vi "CheckParameters.vi"(8 "error in (no error)":errorcluster, 10 "Parameters":u32[](array[numeric]), 11 "HF-Felder in":refnum<class "HF-Felder.lvclass">) -> (0 "error out":errorcluster, 3 "HF-Felder out":refnum<class "HF-Felder.lvclass">)   [LabVIEW 2013, in "HF-Felder.lvclass"]
uses:
  HF-Felder.lvclass
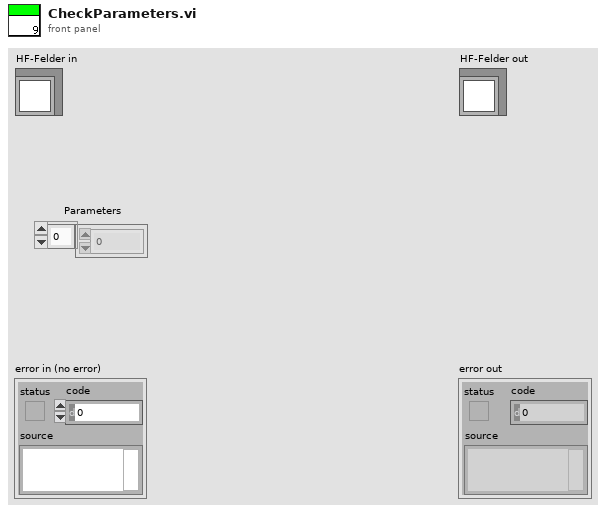
[diagram p1: front panel]
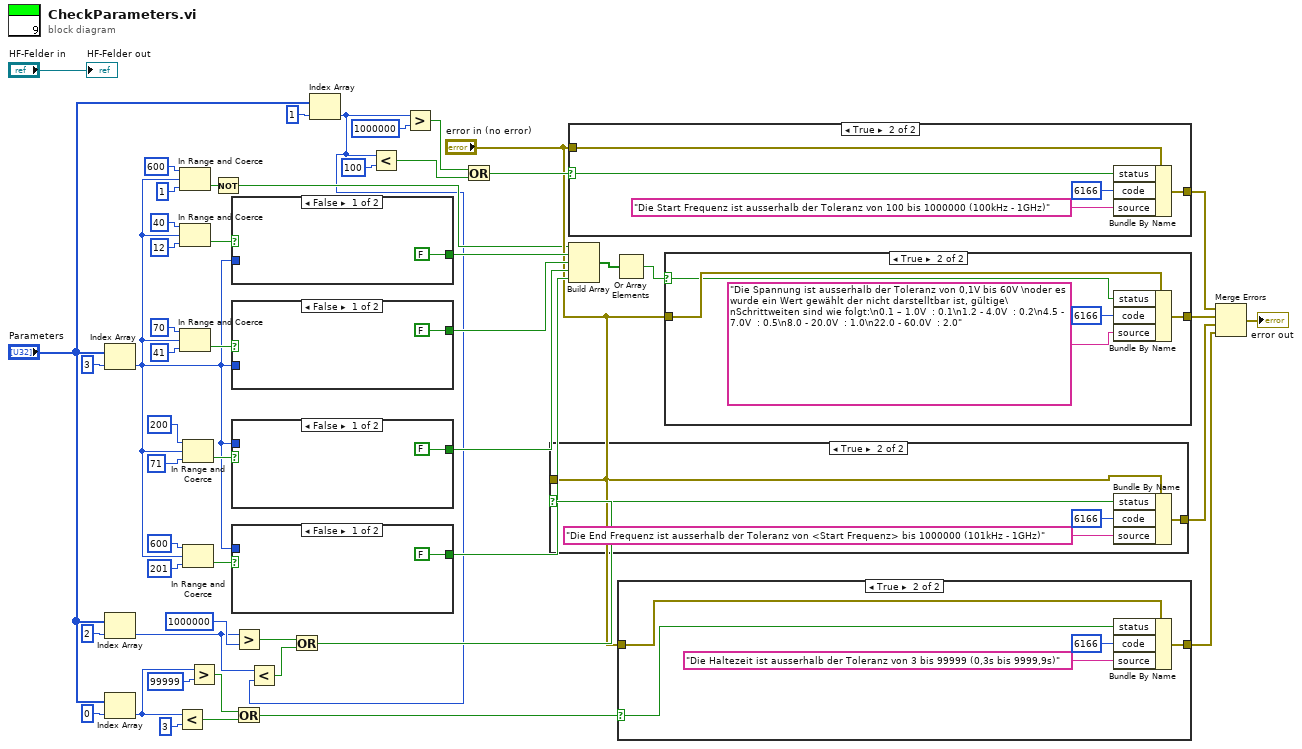
[diagram p0: block diagram]
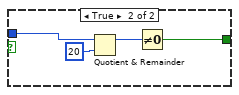
[diagram p2: hidden frame]
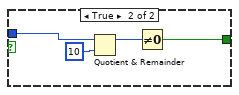
[diagram p3: hidden frame]
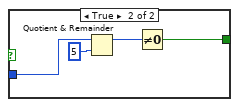
[diagram p4: hidden frame]
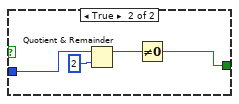
[diagram p5: hidden frame]
diagram:
  n1 = Index Array(array="Parameters", index=3) -> (element=w4:u32)
  n2 = Index Array(array="Parameters", index=2) -> (element=w30:u32)
  n3 = Index Array(array="Parameters", index=0) -> (element=w29:u32)
  n4 = Less?(x=w29, y=u32 3) -> (x < y?=w43:bool)
  n5 = In Range and Coerce(upper limit=u32 600 ("Obergrenze"), x=w4, lower limit=u32 1 ("Untergrenze")) -> (In Range?=w3:bool)  [unwired: 1 out]
  n6 = In Range and Coerce(upper limit=u32 40 ("Obergrenze"), x=w4, lower limit=u32 12 ("Untergrenze")) -> (In Range?=w21:bool)  [unwired: 1 out]
  n7 = In Range and Coerce(upper limit=u32 70 ("Obergrenze"), x=w4, lower limit=u32 41 ("Untergrenze")) -> (In Range?=w15:bool)  [unwired: 1 out]
  n8 = In Range and Coerce(upper limit=u32 200 ("Obergrenze"), x=w4, lower limit=u32 71 ("Untergrenze")) -> (In Range?=w14:bool)  [unwired: 1 out]
  n9 = In Range and Coerce(upper limit=u32 600 ("Obergrenze"), x=w4, lower limit=u32 201 ("Untergrenze")) -> (In Range?=w13:bool)  [unwired: 1 out]
  n10 = Greater?(x=w29, y=u32 99999) -> (0:w44:bool)
  n11 = Not(x=w3) -> (.not. x?=w2:bool)
  n12 = case shown="False" w21 {
    tunnel: w4 -> [_ w57]
    tunnel: [FALSE w54] -> w18
    frame False {
    }
    frame True {
      n13 = Quotient & Remainder(x=w57, y=u32 2) -> (x-y*floor(x/y)=w55:u32)  [unwired: 1 out]
      n14 = Not Equal To 0?(x=w55) -> (x != 0?=w54:bool)
    }
  }
  n15 = case shown="False" w15 {
    tunnel: w4 -> [_ w62]
    tunnel: [FALSE w59] -> w12
    frame False {
    }
    frame True {
      n16 = Quotient & Remainder(x=w62, y=u32 5) -> (x-y*floor(x/y)=w60:u32)  [unwired: 1 out]
      n17 = Not Equal To 0?(x=w60) -> (x != 0?=w59:bool)
    }
  }
  n18 = case shown="False" w14 {
    tunnel: w4 -> [_ w67]
    tunnel: [FALSE w64] -> w11
    frame False {
    }
    frame True {
      n19 = Quotient & Remainder(x=w67, y=u32 10) -> (x-y*floor(x/y)=w65:u32)  [unwired: 1 out]
      n20 = Not Equal To 0?(x=w65) -> (x != 0?=w64:bool)
    }
  }
  n21 = case shown="False" w13 {
    tunnel: w4 -> [_ w72]
    tunnel: [FALSE w69] -> w10
    frame False {
    }
    frame True {
      n22 = Quotient & Remainder(x=w72, y=u32 20) -> (x-y*floor(x/y)=w70:u32)  [unwired: 1 out]
      n23 = Not Equal To 0?(x=w70) -> (x != 0?=w69:bool)
    }
  }
  n24 = Greater?(x=w30, y=u32 1000000) -> (0:w41:bool)
  n25 = Or(x=w44, y=w43) -> (x .or. y?=w47:bool)
  n26 = Index Array(array="Parameters", index=1) -> (element=w1:u32)
  n27 = Less?(x=w30, y=w1) -> (x < y?=w40:bool)
  n28 = Or(x=w41, y=w40) -> (x .or. y?=w48:bool)
  n29 = Less?(x=w1, y=u32 100) -> (x < y?=w36:bool)
  n30 = Greater?(x=w1, y=u32 1000000) -> (0:w37:bool)
  n31 = Or(x=w37, y=w36) -> (x .or. y?=w46:bool)
  n32 = case shown="True" w48 {
    selector: w48 -> [_ w77]
    tunnel: "error in (no error)" -> [w73 w78]
    tunnel: [w73 w74] -> w51
    frame False {
    }
    frame True {
      n33 = Bundle By Name(cluster=w78, "status"=w77, "code"=6166, "source"="Die End Frequenz ist ausserhalb der Toleranz von <Start Frequenz> bis 1000000 (101kHz - 1GHz)") -> (w74:errorcluster)
    }
  }
  n34 = case shown="True" w46 {
    selector: w46 -> [_ w83]
    tunnel: "error in (no error)" -> [w79 w84]
    tunnel: [w79 w80] -> w49
    frame False {
    }
    frame True {
      n35 = Bundle By Name(cluster=w84, "status"=w83, "code"=6166, "source"="Die Start Frequenz ist ausserhalb der Toleranz von 100 bis 1000000 (100kHz - 1GHz)") -> (w80:errorcluster)
    }
  }
  n36 = Build Array(w2, w18, w12, w11, w10) -> (w17:bool[])
  n37 = Or Array Elements(Boolean array=w17) -> (logical OR=w16:bool)
  n38 = case shown="True" w47 {
    selector: w47 -> [_ w90]
    tunnel: [w85 w87] -> w52
    tunnel: "error in (no error)" -> [w85 w86]
    frame False {
    }
    frame True {
      n39 = Bundle By Name(cluster=w86, "status"=w90, "code"=6166, "source"="Die Haltezeit ist ausserhalb der Toleranz von 3 bis 99999 (0,3s bis 9999,9s)") -> (w87:errorcluster)
    }
  }
  n40 = case shown="True" w16 {
    selector: w16 -> [_ w95]
    tunnel: "error in (no error)" -> [w91 w96]
    tunnel: [w91 w92] -> w50
    frame False {
    }
    frame True {
      n41 = Bundle By Name(cluster=w96, "status"=w95, "code"=6166, "source"="Die Spannung ist ausserhalb der Toleranz von 0,1V bis 60V \noder es wurde ein Wert gewählt der nicht darstelltbar ist, gültige\nSchrittweiten sind wie folgt:\n0.1 – 1.0V  : 0.1\n1.2 - 4.0V  : 0.2\n4.5 - 7.0V  : 0.5\n8.0 - 20.0V  : 1.0\n22.0 - 60.0V  : 2.0") -> (w92:errorcluster)
    }
  }
  n42 = Merge Errors(w49, w50, w51, w52) -> (→"error out":errorcluster)
  "HF-Felder out" <- "HF-Felder in"
